vi "Accumulator.vi"(11 "in":dbl) -> (3 "accumulate_out":dbl)   [LabVIEW 2020]
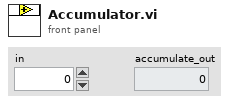
[diagram p1: front panel]
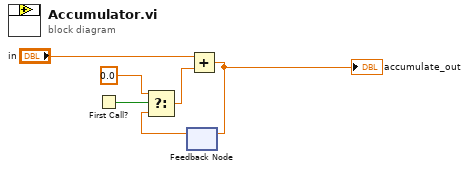
[diagram p0: block diagram]
diagram:
  n1 = First Call?() -> (First Call?: T/F=w3:bool)
  n2 = feedback #1() -> (w1:dbl)  [unwired: 1 in]
  n3 = Select(t=0.0 ("f"), s=w3, f=w1) -> (s? t:f=w2:dbl)
  n4 = Add(x="in", y=w2) -> (x+y=w5:dbl)
  "accumulate_out" <- w5
  n5 = feedback-in #1(w5) -> ()
